vi "onTestDiscovery.vi"(8 "error in (no error)":errorcluster, 11 "Test Runner.Project in":refnum<class "Test Runner.Class.lvclass">) -> (0 "error out":errorcluster, 2 "Tests VIs":path[](array[path]), 3 "Test Runner.Project out":refnum<class "Test Runner.Class.lvclass">)   [LabVIEW 2013, in "Caraya.lvlib" / "Test Runner.Class.lvclass"]
uses:
  Test Runner.Class.lvclass
  Test Runner.Class.lvclass/Test Runner.Class.ctl
  Test Runner/Test Runner.lvclass
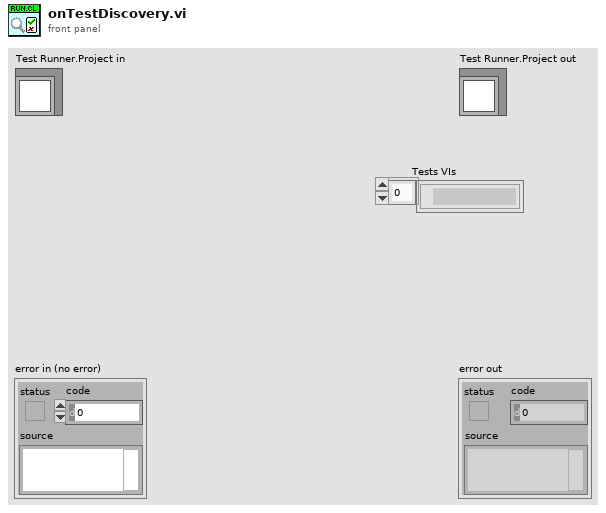
[diagram p1: front panel]
types:
  T1 = enum32{"invalid scope", "public", "private", "protected", "community"}
  T2 = typedef "NI_FileType.lvlib/LVFileType.ctl" = enum32{"Invalid file", "Unknown type", "Instrument", "Control", "Polymorphic VI", "Project", "Library", "LVClass", "XControl", "XNode", "Shared library", ".NET assembly", "ActiveX interface", "CIN", "Run-time menu", "Palette menu", "Help file", "LLB", "XNode Edit Dependency", "Class Private Data Control", "Statechart", "MathScript .m file", "Ladder Diagram", "LVLibp"}
  T3 = cluster{"path":path, "delimited name":string, "type":T2, "iState":u32, "iStyle":u16, "wStyle":u16, "buttons":u16, "viflags":u32, "viflags2":u32, "links":u32[]}[]
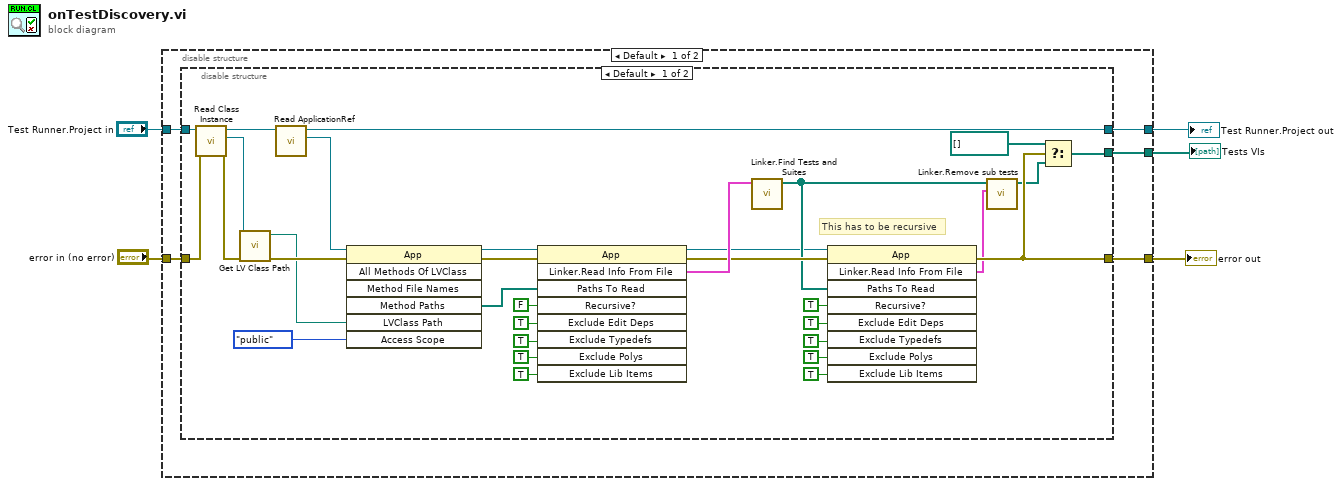
[diagram p0: block diagram]
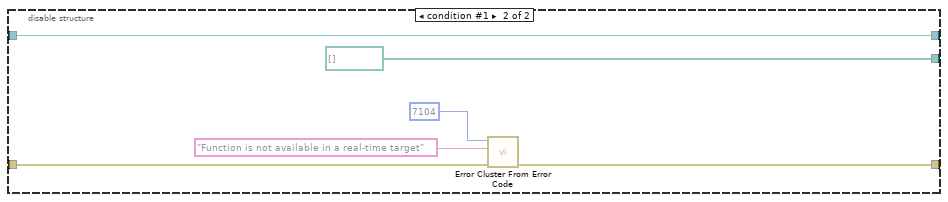
[diagram p2: hidden frame]
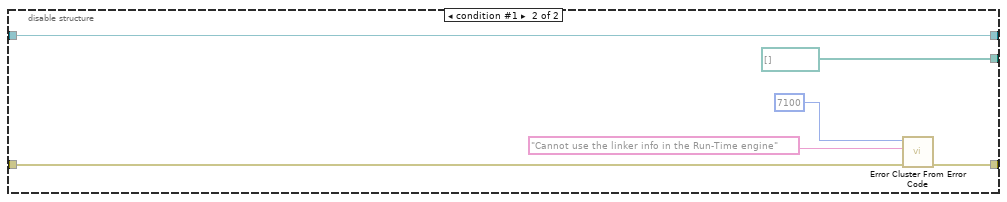
[diagram p3: hidden frame]
diagram:
  n1 = disable-structure shown="Default" {
    disable-tunnel: [w10 w52] -> w2
    disable-tunnel: "Test Runner.Project in" -> [w6 w51]
    disable-tunnel: [w9 w51] -> w3
    disable-tunnel: [w8 path[] [] ("Test VIs")] -> w1
    disable-tunnel: "error in (no error)" -> [w7 w49]
    frame condition #0 (active) {
      n2 = disable-structure shown="Default" {
        disable-tunnel: [w42 w44] -> w10
        disable-tunnel: [w11 w48] -> w9
        disable-tunnel: [w41 path[] [] ("Test VIs")] -> w8
        disable-tunnel: w7 -> [w40 w45]
        disable-tunnel: w6 -> [w39 w48]
        frame condition #0 (active) {
          # "This has to be recursive"
          n3 = call "Read Class Instance.vi"("error in (no error)"=w40, "Test Runner.Project in"=w39) -> ("error out"=w20:errorcluster, "Instance"=w21:refnum<class>, "Test Runner.Project out"=w12:refnum<class "Test Runner.Class.lvclass">)  [unwired: 7 in]
          n4 = call <vilib>:"Get LV Class Path.vi"("error in (no error)"=w20, "object"=w21) -> ("error out"=w19:errorcluster, "class path"=w16:path)  [unwired: 8 in]
          n5 = call "Read ApplicationRef.vi"("Test Runner in"=w12) -> ("Application"=w15:refnum<vi>, "Test Runner out"=w11:refnum<class "Test Runner.Class.lvclass">)  [unwired: 8 in, 1 out]
          n6 = invoke class="App" method="All Methods Of LVClass"(reference=w15, error in=w19, "LVClass Path"=w16, "Access Scope"=T1."public") -> (reference out=w14:refnum<vi>, error out=w18:errorcluster, "Method Paths"=w17:path[])  [unwired: 3 in, 4 out]
          n7 = invoke class="App" method="Linker.Read Info From File"(reference=w14, error in=w18, "Paths To Read"=w17, "Recursive?"=FALSE, "Exclude Edit Deps"=TRUE ("Exclude Edit Time Dependencies"), "Exclude Typedefs"=TRUE, "Exclude Polys"=TRUE ("Exclude Poly VIs"), "Exclude Lib Items"=TRUE ("Exclude Unused Library Items")) -> (reference out=w13:refnum<vi>, error out=w25:errorcluster, "Linker.Read Info From File"=w32:T3)  [unwired: 1 in, 6 out]
          n8 = call "Linker.Find Tests and Suites.vi"("Linker:Read Info From File"=w32) -> ("All VIs defining a test (excluding those defining a suite)"=w23:path[])  [unwired: 8 in, 2 out]
          n9 = invoke class="App" method="Linker.Read Info From File"(reference=w13, error in=w25, "Paths To Read"=w23, "Recursive?"=TRUE, "Exclude Edit Deps"=TRUE ("Exclude Edit Time Dependencies"), "Exclude Typedefs"=TRUE, "Exclude Polys"=TRUE ("Exclude Poly VIs"), "Exclude Lib Items"=TRUE ("Exclude Unused Library Items")) -> (error out=w42:errorcluster, "Linker.Read Info From File"=w24:T3)  [unwired: 1 in, 7 out]
          n10 = call "Linker.Remove sub tests.vi"("Linker.Read Info From File"=w24, "Tests"=w23) -> ("Array"=w31:path[])  [unwired: 9 in]
          n11 = Select(t=path[] [], s=w42, f=w31) -> (s? t:f=w41:path[])
        }
        frame condition #1 {
          n12 = call <vilib>:"Error Cluster From Error Code.vi"("error in (no error)"=w45, "error message (\"\")"="Function is not available in a real-time target" ("error message (\"\")"), "error code (0)"=7104) -> ("error out"=w44:errorcluster)  [unwired: 6 in]
        }
      }
    }
    frame condition #1 {
      n13 = call <vilib>:"Error Cluster From Error Code.vi"("error in (no error)"=w49, "error message (\"\")"="Cannot use the linker info in the Run-Time engine" ("error message (\"\")"), "error code (0)"=7100) -> ("error out"=w52:errorcluster)  [unwired: 6 in]
    }
  }
  "error out" <- w2
  "Test Runner.Project out" <- w3
  "Tests VIs" <- w1
